vi "update_attrs.vi"(8 "error in (no error)":errorcluster, 10 "Nested Enqueuers Map":T1(c390), 11 "root_actor in":refnum<class "root_actor.lvclass">) -> (0 "error out":errorcluster, 3 "root_actor out":refnum<class "root_actor.lvclass">)   [LabVIEW 2025, in "root_actor.lvlib" / "root_actor.lvclass"]
uses:
  root_actor.lvclass
  <vilib>/ActorFramework/Message Enqueuer/Message Enqueuer.lvclass
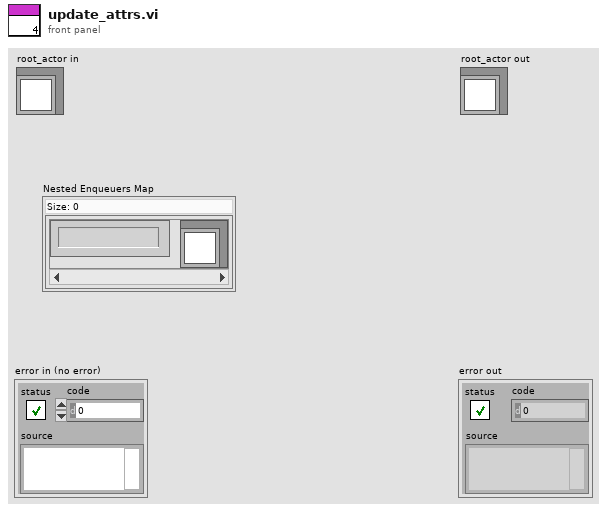
[diagram p1: front panel]
types:
  T1 = map{string, refnum<class "Message Enqueuer.lvclass">}
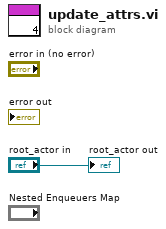
[diagram p0: block diagram]
diagram:
  "root_actor out" <- "root_actor in"
